vi "strain_test2.vi"() -> ()   [LabVIEW 2014]
uses:
  <vilib>/LabVIEW Targets/FPGA/cRIO/shared/nicrio_ModuleControls/nicrio_cRIO-9237_DataRatesRing.ctl
  <vilib>/LabVIEW Targets/FPGA/cRIO/shared/nicrio_ModuleControls/nicrio_cRIO-9237_ExcitationVoltageRing.ctl
  <vilib>/rvi/Emulation/niFpgaGetClockAttributes.vi
  <vilib>/rvi/Emulation/niFpgaSctlEmulationGetInTimedLoop.vi
  <vilib>/rvi/Emulation/niFpgaEmulationReportErrorSimple.vi
  <vilib>/rvi/eio/common/nirviEmuTemplatePropertySet_errors.vi
  <vilib>/rvi/eio/common/nirviEmuTemplateMethod_errors.vi
  <vilib>/rvi/Emulation/niFpgaProcessEmulError.vi
  <vilib>/rvi/Emulation/niFpgaCriticalErrorInLSC.vi
  <vilib>/eio/EIOPropertyNode/EIOPropertyNode.xnode
  <vilib>/eio/EIONode/EIONode.xnode
  <vilib>/rvi/eio/common/nirviEmuTemplatePropertyGet_errors.vi
  <vilib>/rvi/eio/common/nirviEmuTemplatePropertyGet_noerrors.vi
  <vilib>/rvi/eio/common/nirviEmuTemplatePropertySet_noerrors.vi
panel:
  in  "Stop":bool
  out "Mod6/AI2":fxp<+/-,24,-4>
  in  "Shunt Cal Enable":bool
  in  "Half-Bridge Enable":bool
  in  "Excitation Voltage":T1 items=["2.5 Volts", "3.3 Volts", "5.0 Volts", "10.0 Volts", "External Excitation"]
  in  "Data Rate":T2=1 items=["50.000 kS/s (NI 9237)"=1, "25.000 kS/s (NI 9237)"=2, "16.667 kS/s (NI 9237)"=3, "12.500 kS/s (NI 9237)"=4, "10.000 kS/s (NI 9237)"=5, "8.333 kS/s (NI 9237)"=6, "7.143 kS/s (NI 9237)"=7, "6.250 kS/s (NI 9237)"=8, "5.556 kS/s (NI 9237)"=9, "5.000 kS/s (NI 9237)"=10, "4.545 kS/s (NI 9237)"=11, "4.167 kS/s (NI 9237)"=12, "3.846 kS/s (NI 9237)"=13, "3.571 kS/s (NI 9237)"=14, "3.333 kS/s (NI 9237)"=15, "3.125 kS/s (NI 9237)"=16, "2.941 kS/s (NI 9237)"=17, "2.778 kS/s (NI 9237)"=18, "2.632 kS/s (NI 9237)"=19, "2.500 kS/s (NI 9237)"=20, "2.381 kS/s (NI 9237)"=21, "2.273 kS/s (NI 9237)"=22, "2.174 kS/s (NI 9237)"=23, "2.083 kS/s (NI 9237)"=24, "2.000 kS/s (NI 9237)"=25, "1.923 kS/s (NI 9237)"=26, "1.852 kS/s (NI 9237)"=27, "1.786 kS/s (NI 9237)"=28, "1.724 kS/s (NI 9237)"=29, "1.667 kS/s (NI 9237)"=30, "1.613 kS/s (NI 9237)"=31]
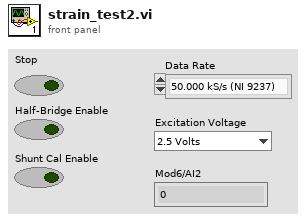
[diagram p1: front panel]
types:
  T1 = typedef "nicrio_cRIO-9237_ExcitationVoltageRing.ctl" = u8
  T2 = typedef "nicrio_cRIO-9237_DataRatesRing.ctl" = u8
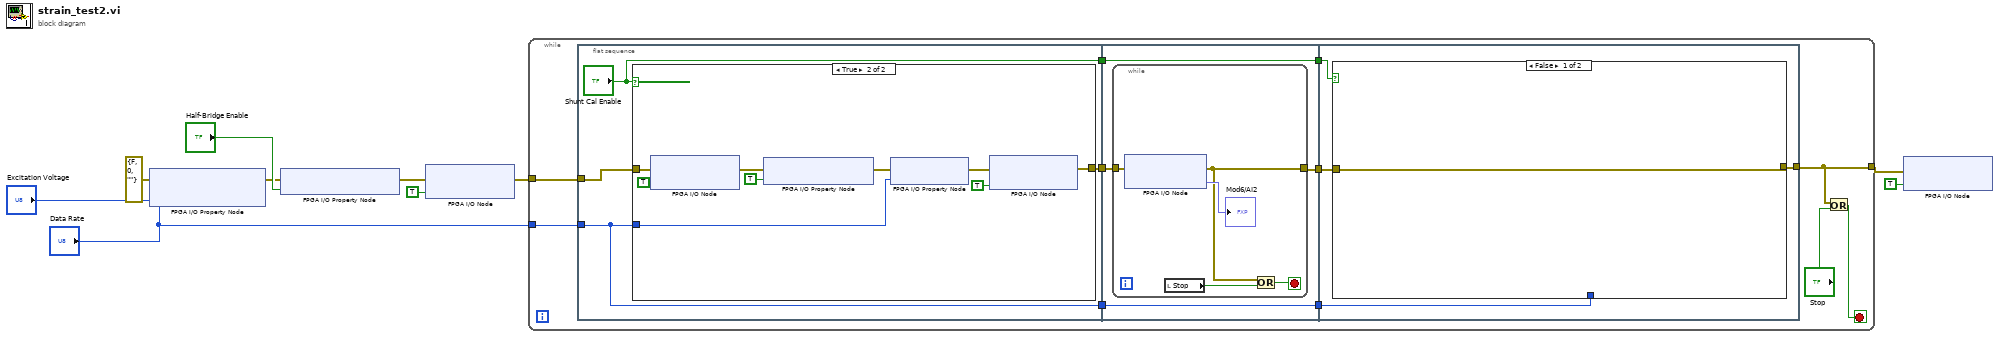
[diagram p0: block diagram]
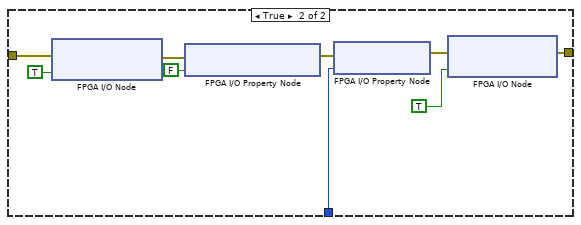
[diagram p3: hidden frame]
diagram:
  n1 = xnode "FPGA I/O Property Node"("error in"=errorcluster {"status"=FALSE, "code"=0, "source"=""}, "Data Rate"="Data Rate", "Excitation Voltage"="Excitation Voltage") -> ("error out"=w7:errorcluster)  [unwired: 1 in, 1 out]
  n2 = xnode "FPGA I/O Property Node"("error in"=w7, "Half-Bridge Enable"="Half-Bridge Enable") -> ("error out"=w6:errorcluster)  [unwired: 1 in, 1 out]
  n3 = xnode "FPGA I/O Node"("error in"=w6, "Mod6/Start"=TRUE) -> ("error out"=w4:errorcluster)  [unwired: 1 in, 1 out]
  n4 = while {
    tunnel: w4 -> [w21]
    tunnel: "Data Rate" -> [w20]
    tunnel: [w12] -> w2
    stop <- w13 stop-if-true
    n5 = flat-sequence {
      tunnel: w21 -> [w25]
      tunnel: w20 -> [w24]
      tunnel: [w24] -> w19
      tunnel: ["Shunt Cal Enable"] -> w18
      tunnel: [w22] -> w17
      tunnel: w19 -> [w36]
      tunnel: w18 -> [w38]
      tunnel: w17 -> [w39]
      tunnel: [w38] -> w16
      tunnel: [w37] -> w15
      tunnel: [w36] -> w14
      tunnel: w16 -> [w48]
      tunnel: w15 -> [w47]
      tunnel: w14 -> [w46]
      tunnel: [w45] -> w12
      frame #0 {
        n6 = case shown="True" "Shunt Cal Enable" {
          tunnel: w25 -> [w26 w33]
          tunnel: w24 -> [_ w31]
          tunnel: [w26 w28] -> w22
          frame False {
          }
          frame True {
            n7 = xnode "FPGA I/O Node"("error in"=w33, "Mod6/Stop"=TRUE) -> ("error out"=w34:errorcluster)  [unwired: 1 in, 1 out]
            n8 = xnode "FPGA I/O Property Node"("error in"=w34, "Shunt Cal Enable"=TRUE) -> ("error out"=w32:errorcluster)  [unwired: 1 in, 1 out]
            n9 = xnode "FPGA I/O Property Node"("error in"=w32, "Data Rate"=w31) -> ("error out"=w30:errorcluster)  [unwired: 1 in, 1 out]
            n10 = xnode "FPGA I/O Node"("error in"=w30, "Mod6/Start"=TRUE) -> ("error out"=w28:errorcluster)  [unwired: 1 in, 1 out]
          }
        }
      }
      frame #1 {
        n11 = while {
          tunnel: w39 -> [w44]
          tunnel: [w40] -> w37
          stop <- w41 stop-if-true
          n12 = xnode "FPGA I/O Node"("error in"=w44) -> ("error out"=w40:errorcluster, "Mod6/AI2"=→"Mod6/AI2":fxp<+/-,24,-4>)  [unwired: 1 in, 1 out]
          n13 = local read "Stop"() -> (w42:bool)
          n14 = Or(x=w40, y=w42) -> (x .or. y?=w41:bool)
        }
      }
      frame #2 {
        n15 = case shown="False" w48 {
          tunnel: w47 -> [w49 w57]
          tunnel: w46 -> [_ w53]
          tunnel: [w49 w50] -> w45
          frame False {
          }
          frame True {
            n16 = xnode "FPGA I/O Node"("error in"=w57, "Mod6/Stop"=TRUE) -> ("error out"=w55:errorcluster)  [unwired: 1 in, 1 out]
            n17 = xnode "FPGA I/O Property Node"("error in"=w55, "Shunt Cal Enable"=FALSE) -> ("error out"=w54:errorcluster)  [unwired: 1 in, 1 out]
            n18 = xnode "FPGA I/O Property Node"("error in"=w54, "Data Rate"=w53) -> ("error out"=w52:errorcluster)  [unwired: 1 in, 1 out]
            n19 = xnode "FPGA I/O Node"("error in"=w52, "Mod6/Start"=TRUE) -> ("error out"=w50:errorcluster)  [unwired: 1 in, 1 out]
          }
        }
      }
    }
    n20 = Or(x=w12, y="Stop") -> (x .or. y?=w13:bool)
  }
  n21 = xnode "FPGA I/O Node"("error in"=w2, "Mod6/Stop"=TRUE) -> ()  [unwired: 1 in, 2 out]
